vi "Read Loop.vi"(8 "error in (no error)":errorcluster, 11 "WAMP Client in":refnum<class "WAMP Client.lvclass">) -> (0 "error out":errorcluster, 3 "WAMP Client out":refnum<class "WAMP Client.lvclass">)   [LabVIEW 2020, in "wamplv.lvlib" / "WAMP Client.lvclass"]
uses:
  WAMP Client.lvclass
  WAMP Client.lvclass/WAMP Client.ctl
  TypeDef/Internal Message Type.ctl
  TypeDef/Internal Message.ctl
  TypeDef/Termination Reason Enum.ctl
  <vilib>/JDP Science/JSONtext/Get Array Elements.vi
  <vilib>/Utility/error.llb/Error Cluster From Error Code.vi
  <vilib>/ErrorRing/Error Ring.xnode
  Private/Comm Handlers/ICommHandler/ICommHandler.lvclass
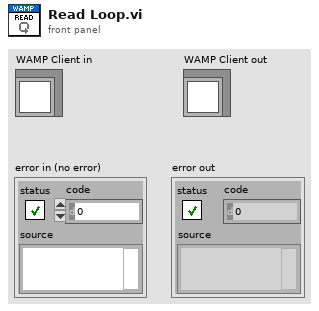
[diagram p1: front panel]
types:
  T1 = typedef "wamplv.lvlib/WAMP Client.lvclass/Internal Message Type.ctl" = enum16{"Subscribe", "Handle Subscribed", "Handle Event", "Unsubscribe", "Handle Unsubscribed", "Publish", "Handled Published", "Goodbye", "Handle Goodbye", "Call", "Handle Result", "Register", "Handle Registered", "Unregister", "Handle Unregistered", "Handle Invocation", "Yield", "Error"}
  T2 = typedef "wamplv.lvlib/WAMP Client.lvclass/Internal Message.ctl" = cluster{"Internal Message Type":T1, "Variant":variant}
  T3 = typedef "wamplv.lvlib/WAMP Client.lvclass/Termination Reason Enum.ctl" = enum16{"Goodbye Received", "Abort Received", "Send Goodbye", "Send Abort", "Read Loop Failure", "Write Loop Failure", "Message Loop Failure"}
  T4 = typedef "wamplv.lvlib/WAMP Client.lvclass/WAMP Message Codes.ctl" = u16
  T5 = typedef "wamplv.lvlib/WAMP Client.lvclass/WAMP Received Message.ctl" = cluster{"Message JSON":string[], "Message Codes":T4}
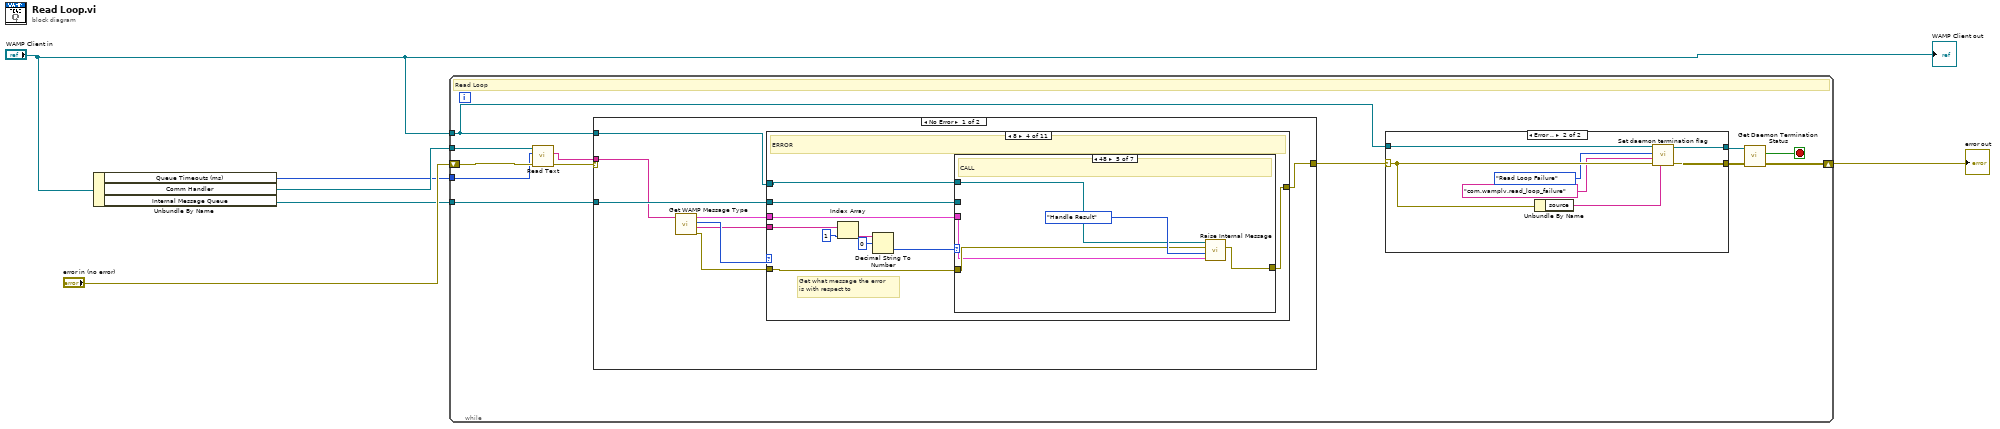
[diagram p0: block diagram]
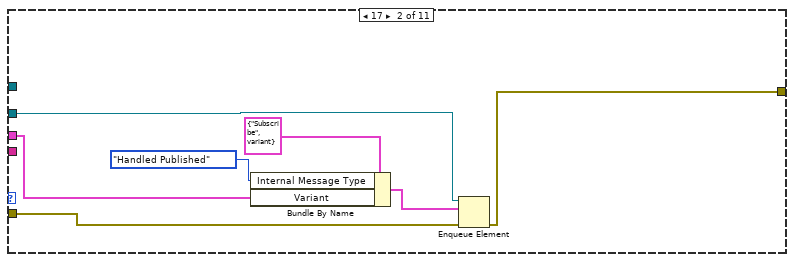
[diagram p3: hidden frame]
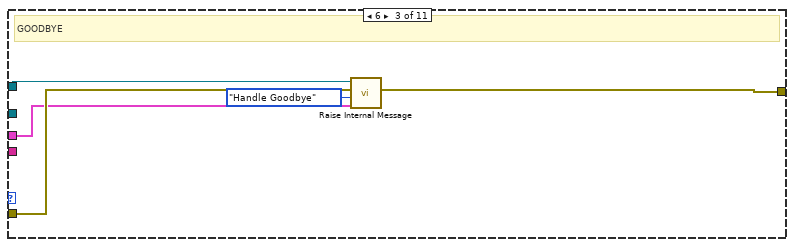
[diagram p4: hidden frame]
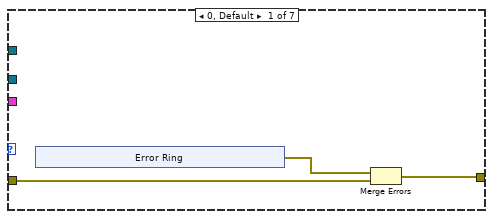
[diagram p5: hidden frame]
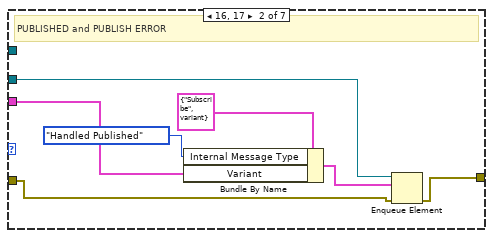
[diagram p6: hidden frame]
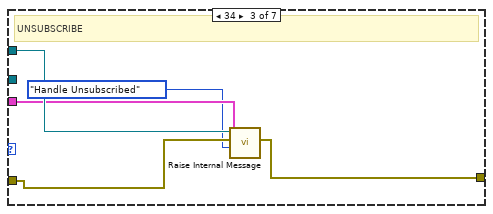
[diagram p7: hidden frame]
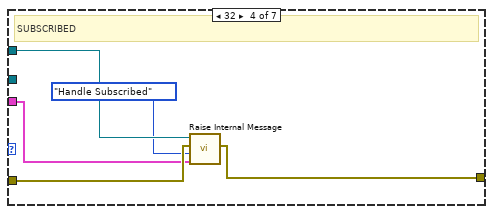
[diagram p8: hidden frame]
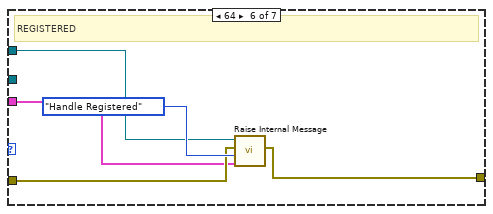
[diagram p9: hidden frame]
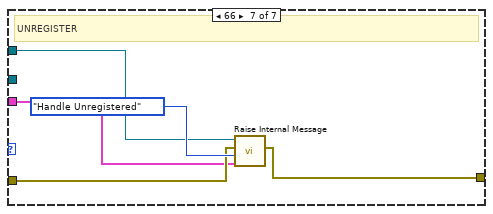
[diagram p10: hidden frame]
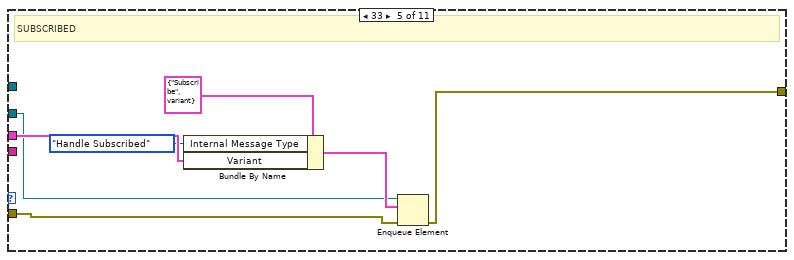
[diagram p11: hidden frame]
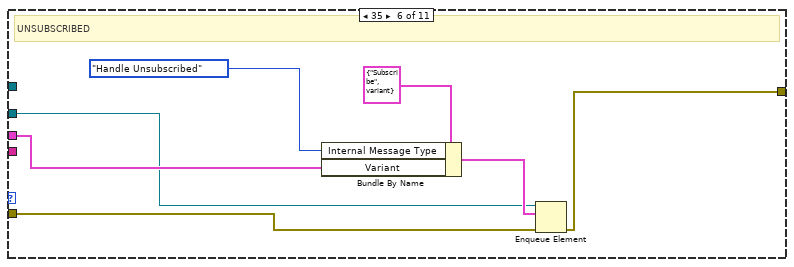
[diagram p12: hidden frame]
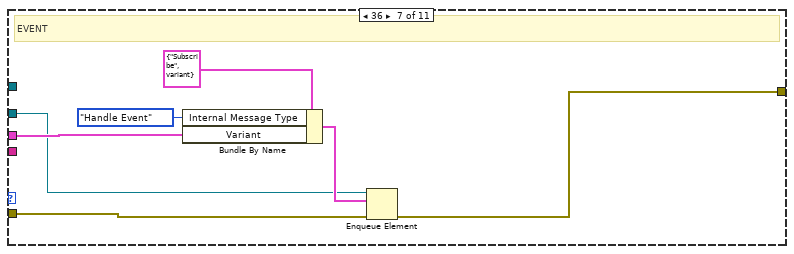
[diagram p13: hidden frame]
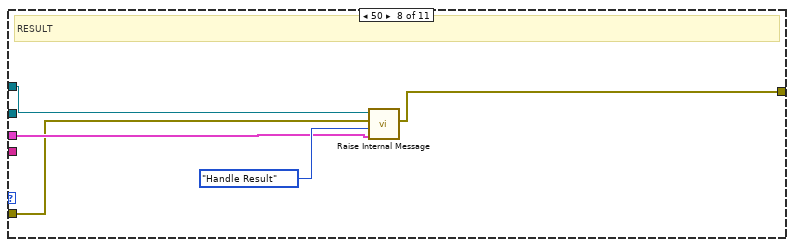
[diagram p14: hidden frame]
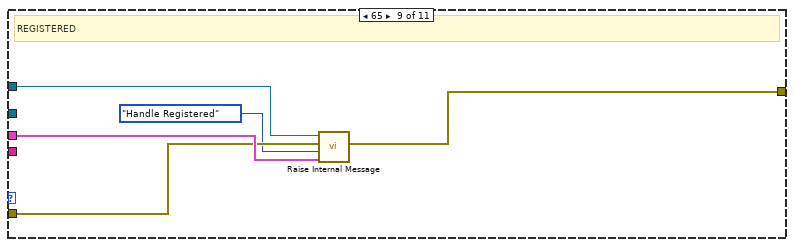
[diagram p15: hidden frame]
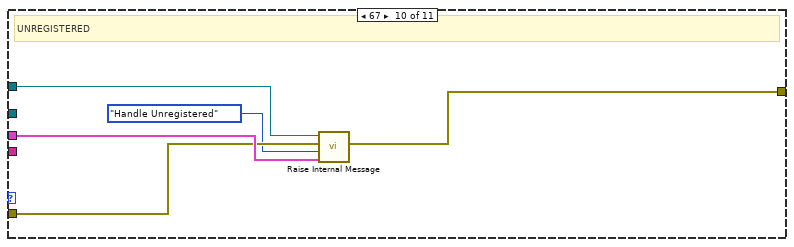
[diagram p16: hidden frame]
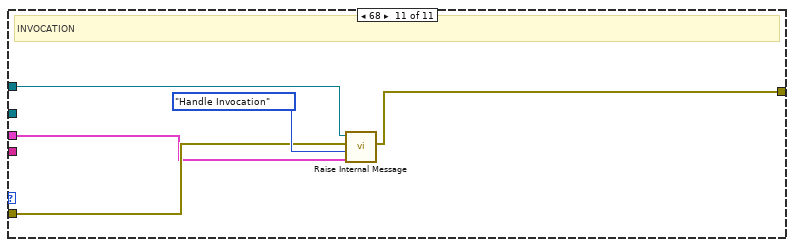
[diagram p17: hidden frame]
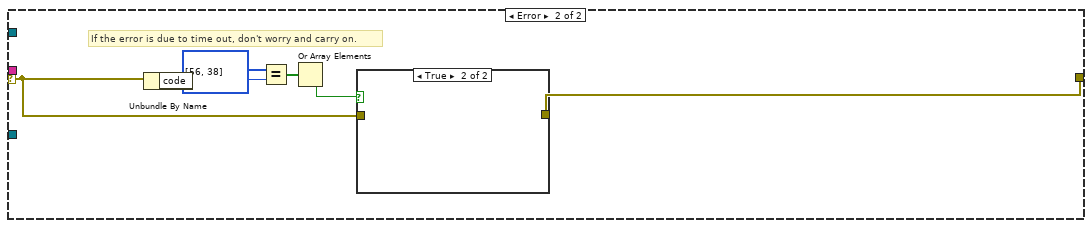
[diagram p18: hidden frame]
diagram:
  n1 = Unbundle By Name("WAMP Client in") -> ("Queue Timeouts (ms)"=w1:i32, "Comm Handler"=w5:refnum<class "ICommHandler.lvclass">, "Internal Message Queue"=w3:refnum<queue>)
  n2 = while {
    shift-right: [w12] -> w4
    shift-left: "error in (no error)" -> [w10]
    tunnel: w5 -> [w18]
    tunnel: w3 -> [w17]
    tunnel: "WAMP Client in" -> [w11]
    tunnel: w1 -> [w9]
    stop <- w13 stop-if-true
    # "Read Loop"
    n3 = call-dynamic "Read Text.vi"("error in (no error)"=w10, "timeout ms (1000)"=w9, "ICommHandler in"=w18) -> ("error out"=w8:errorcluster, "String"=w7:string)  [unwired: 4 in, 1 out]
    n4 = case shown="No Error" w8 {
      selector: w8 -> [_ w135]
      tunnel: [w25 w134] -> w16
      tunnel: w7 -> [w22 _]
      tunnel: w17 -> [w24 _]
      tunnel: w11 -> [w23 _]
      frame No Error {
        n5 = call "Get WAMP Message Type.vi"("JSON"=w22) -> ("error out"=w20:errorcluster, "<JSON>"=w19:string[], "Message Codes"=w21:T4, "WAMP Message"=w26:T5)  [unwired: 7 in]
        n6 = case shown="8" w21 {
          tunnel: w19 -> [_ _ _ w46 _ _ _ _ _ _ _]
          tunnel: w20 -> [w27 w30 w38 w44 w91 w98 w106 w112 w117 w122 w127]
          tunnel: w26 -> [_ w31 w36 w45 w93 w100 w107 w113 w118 w123 w125]
          tunnel: [w27 w29 w35 w43 w92 w99 w105 w111 w116 w121 w126] -> w25
          tunnel: w24 -> [_ w28 _ w41 w89 w96 w103 _ _ _ _]
          tunnel: w23 -> [_ _ w39 w40 _ _ _ w110 w119 w124 w129]
          frame 0, Default {
          }
          frame 17 {
            n7 = Bundle By Name(cluster=T2 {"Internal Message Type"=enum."Subscribe", "Variant"=variant} ("Cluster"), "Internal Message Type"=Internal_Message_Type."Handled Published", "Variant"=w31) -> (w33:T2)
            n8 = Enqueue Element(queue=w28, element=w33, error in (no error)=w30) -> (error out=w29:errorcluster)  [unwired: 1 in, 2 out]
          }
          frame 6 {
            # "GOODBYE"
            n9 = call "Raise Internal Message.vi"("Variant"=w36, "Internal Message Type"=Internal_Message_Type."Handle Goodbye", "error in (no error)"=w38, "WAMP Client in"=w39) -> ("error out"=w35:errorcluster)  [unwired: 6 in, 1 out]
          }
          frame 8 {
            # "Get what message the error \nis with respect to"
            # "ERROR"
            n10 = Index Array(array=w46, index=1) -> (element=w48:string)
            n11 = Decimal String To Number(string=w48, offset=0) -> (number=w47:i32)  [unwired: 1 in, 1 out]
            n12 = case shown="48" w47 {
              tunnel: w45 -> [_ w59 w65 w70 w76 w79 w84]
              tunnel: w44 -> [w51 w60 w66 w73 w77 w81 w86]
              tunnel: [w52 w58 w68 w72 w74 w80 w85] -> w43
              tunnel: w41 -> [_ w57 _ _ _ _ _]
              tunnel: w40 -> [_ _ w67 w71 w75 w82 w87]
              frame 0, Default {
                n13 = xnode "Error Ring"() -> ("error out"=w50:errorcluster)
                n14 = Merge Errors(w50, w51) -> (w52:errorcluster)
              }
              frame 16, 17 {
                # "PUBLISHED and PUBLISH ERROR"
                n15 = Bundle By Name(cluster=T2 {"Internal Message Type"=enum."Subscribe", "Variant"=variant} ("Cluster"), "Internal Message Type"=Internal_Message_Type."Handled Published", "Variant"=w59) -> (w62:T2)
                n16 = Enqueue Element(queue=w57, element=w62, error in (no error)=w60) -> (error out=w58:errorcluster)  [unwired: 1 in, 2 out]
              }
              frame 34 {
                # "UNSUBSCRIBE"
                n17 = call "Raise Internal Message.vi"("Variant"=w65, "Internal Message Type"=Internal_Message_Type."Handle Unsubscribed", "error in (no error)"=w66, "WAMP Client in"=w67) -> ("error out"=w68:errorcluster)  [unwired: 6 in, 1 out]
              }
              frame 32 {
                # "SUBSCRIBED"
                n18 = call "Raise Internal Message.vi"("Variant"=w70, "Internal Message Type"=Internal_Message_Type."Handle Subscribed", "error in (no error)"=w73, "WAMP Client in"=w71) -> ("error out"=w72:errorcluster)  [unwired: 6 in, 1 out]
              }
              frame 48 {
                # "CALL"
                n19 = call "Raise Internal Message.vi"("Variant"=w76, "Internal Message Type"=Internal_Message_Type."Handle Result", "error in (no error)"=w77, "WAMP Client in"=w75) -> ("error out"=w74:errorcluster)  [unwired: 6 in, 1 out]
              }
              frame 64 {
                # "REGISTERED"
                n20 = call "Raise Internal Message.vi"("Variant"=w79, "Internal Message Type"=Internal_Message_Type."Handle Registered", "error in (no error)"=w81, "WAMP Client in"=w82) -> ("error out"=w80:errorcluster)  [unwired: 6 in, 1 out]
              }
              frame 66 {
                # "UNREGISTER"
                n21 = call "Raise Internal Message.vi"("Variant"=w84, "Internal Message Type"=Internal_Message_Type."Handle Unregistered", "error in (no error)"=w86, "WAMP Client in"=w87) -> ("error out"=w85:errorcluster)  [unwired: 6 in, 1 out]
              }
            }
          }
          frame 33 {
            # "SUBSCRIBED"
            n22 = Bundle By Name(cluster=T2 {"Internal Message Type"=enum."Subscribe", "Variant"=variant} ("Cluster"), "Internal Message Type"=Internal_Message_Type."Handle Subscribed", "Variant"=w93) -> (w94:T2)
            n23 = Enqueue Element(queue=w89, element=w94, error in (no error)=w91) -> (error out=w92:errorcluster)  [unwired: 1 in, 2 out]
          }
          frame 35 {
            # "UNSUBSCRIBED"
            n24 = Bundle By Name(cluster=T2 {"Internal Message Type"=enum."Subscribe", "Variant"=variant} ("Cluster"), "Internal Message Type"=Internal_Message_Type."Handle Unsubscribed", "Variant"=w100) -> (w101:T2)
            n25 = Enqueue Element(queue=w96, element=w101, error in (no error)=w98) -> (error out=w99:errorcluster)  [unwired: 1 in, 2 out]
          }
          frame 36 {
            # "EVENT"
            n26 = Bundle By Name(cluster=T2 {"Internal Message Type"=enum."Subscribe", "Variant"=variant} ("Cluster"), "Internal Message Type"=Internal_Message_Type."Handle Event", "Variant"=w107) -> (w108:T2)
            n27 = Enqueue Element(queue=w103, element=w108, error in (no error)=w106) -> (error out=w105:errorcluster)  [unwired: 1 in, 2 out]
          }
          frame 50 {
            # "RESULT"
            n28 = call "Raise Internal Message.vi"("Variant"=w113, "Internal Message Type"=Internal_Message_Type."Handle Result", "error in (no error)"=w112, "WAMP Client in"=w110) -> ("error out"=w111:errorcluster)  [unwired: 6 in, 1 out]
          }
          frame 65 {
            # "REGISTERED"
            n29 = call "Raise Internal Message.vi"("Variant"=w118, "Internal Message Type"=Internal_Message_Type."Handle Registered", "error in (no error)"=w117, "WAMP Client in"=w119) -> ("error out"=w116:errorcluster)  [unwired: 6 in, 1 out]
          }
          frame 67 {
            # "UNREGISTERED"
            n30 = call "Raise Internal Message.vi"("Variant"=w123, "Internal Message Type"=Internal_Message_Type."Handle Unregistered", "error in (no error)"=w122, "WAMP Client in"=w124) -> ("error out"=w121:errorcluster)  [unwired: 6 in, 1 out]
          }
          frame 68 {
            # "INVOCATION"
            n31 = call "Raise Internal Message.vi"("Variant"=w125, "Internal Message Type"=Internal_Message_Type."Handle Invocation", "error in (no error)"=w127, "WAMP Client in"=w129) -> ("error out"=w126:errorcluster)  [unwired: 6 in, 1 out]
          }
        }
      }
      frame Error {
        # "If the error is due to time out, don't worry and carry on."
        n32 = Unbundle By Name(w135) -> ("code"=w133:i32)
        n33 = Equal?(x=i32[] [56, 38] ("y"), y=w133) -> (x = y?=w131:bool[])
        n34 = Or Array Elements(Boolean array=w131) -> (logical OR=w130:bool)
        n35 = case shown="True" w130 {
          tunnel: w135 -> [w136 _]
          tunnel: [w136 _] -> w134
          frame False {
          }
          frame True {
          }
        }
      }
    }
    n36 = case shown="Error .." w16 {
      selector: w16 -> [w138 w143]
      tunnel: [w138 w144] -> w14
      tunnel: [w137 w145] -> w15
      tunnel: w11 -> [w137 w142]
      frame No Error {
      }
      frame Error {
        n37 = Unbundle By Name(w143) -> ("source"=w140:string)
        n38 = call "Set daemon termination flag.vi"("Message"=w140, "error in (no error)"=w143, "Reason URI"="com.wamplv.read_loop_failure", "Reason"=Termination_Reason_Enum."Read Loop Failure" ("Termination Reason"), "WAMP Client (in)"=w142) -> ("error out"=w144:errorcluster, "WAMP Client (out)"=w145:refnum<class "WAMP Client.lvclass">)  [unwired: 5 in]
      }
    }
    n39 = call "Get Daemon Termination Status.vi"("error in (no error)"=w14, "WAMP Client in"=w15) -> ("error out"=w12:errorcluster, "Terminate?"=w13:bool)  [unwired: 6 in, 2 out]
  }
  "error out" <- w4
  "WAMP Client out" <- "WAMP Client in"
